vi "Iteration idx--FGV.vi"(8 "error in (no error)":errorcluster, 11 "Action":enum16{"Reset", "Get", "Increment"}(ring)) -> (0 "error out":errorcluster, 3 "Index":i32)   [LabVIEW 2020]
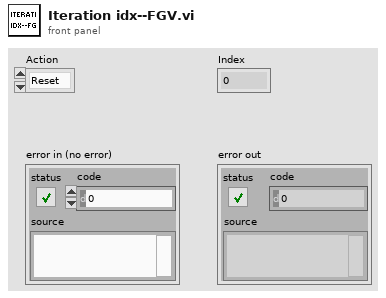
[diagram p1: front panel]
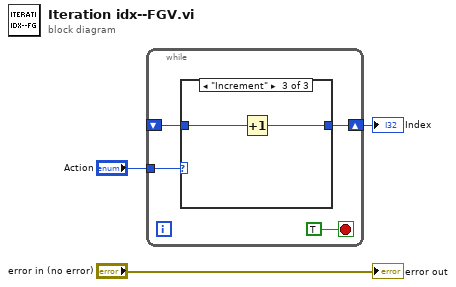
[diagram p0: block diagram]
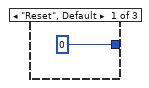
[diagram p2: hidden frame]
diagram:
  n1 = while {
    tunnel: "Action" -> [w6]
    shift-right: [w4] -> w2
    shift-left: _ -> [w5]
    stop <- TRUE stop-if-true
    n2 = case shown="\"Increment\"" w6 {
      tunnel: w5 -> [_ w9 w11]
      tunnel: [0 w9 w10] -> w4
      frame "Reset", Default {
      }
      frame "Get" {
      }
      frame "Increment" {
        n3 = Increment(x=w11) -> (x+1=w10:i32)
      }
    }
  }
  "Index" <- w2
  "error out" <- "error in (no error)"
